vi "relayInternalCommand.vi"(8 "error in (no error)":errorcluster, 11 "DataListenerThisComponent in":refnum<class "DataListenerThisComponent.lvclass">) -> (0 "error out":errorcluster, 3 "DataListenerThisComponent out":refnum<class "DataListenerThisComponent.lvclass">)   [LabVIEW 2015]
uses:
  ComponentTemplateCore/ComponentModel/ComponentModel/DataListener/DataListener.lvclass
  DataListenerThisComponent.lvclass
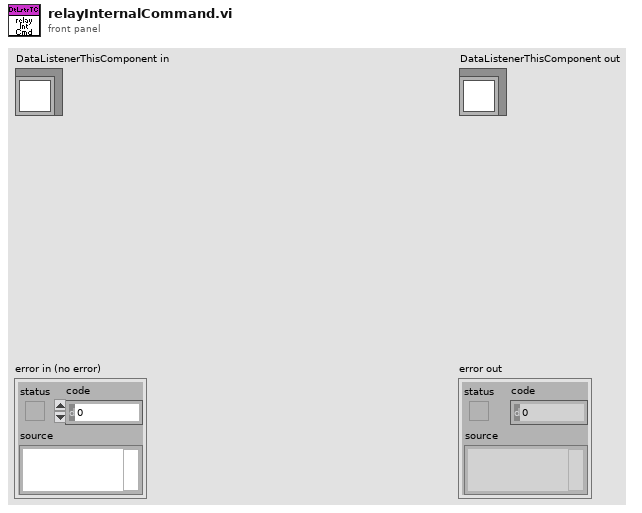
[diagram p1: front panel]
types:
  T1 = typedef "EXATypedefs.lvlib/CommandEvents.ctl" = cluster{"command":refnum<user-event>}
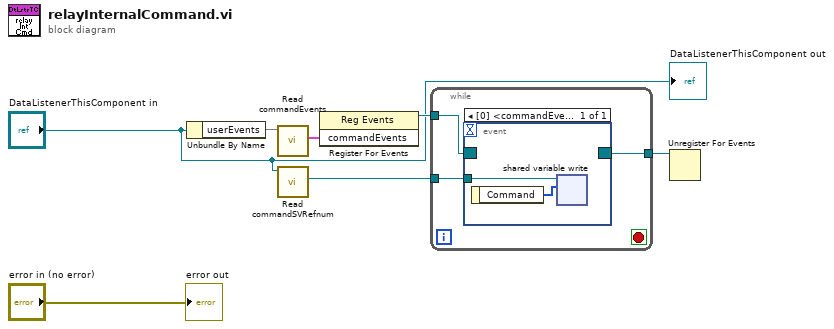
[diagram p0: block diagram]
diagram:
  n1 = Unbundle By Name("DataListenerThisComponent in") -> ("userEvents"=w7)
  n2 = call "Read commandEvents.vi"("UserEventsThisComponent in"=w7) -> ("commandEvents"=w6:T1)  [unwired: 9 in, 1 out]
  n3 = call "Read commandSVRefnum.vi"("DataListener in"="DataListenerThisComponent in") -> ("commandSVRefnum"=w4:refnum<k21>)  [unwired: 9 in, 1 out]
  n4 = register-events(w6) -> (reference out=w5:refnum<event-registration>)  [unwired: 2 in, 1 out]
  n5 = while {
    tunnel: w5 -> [w10]
    tunnel: w4 -> [w9]
    tunnel: [w8] -> w3
    stop <- _ stop-if-true
    n6 = event shown="[0] <commandEvents.command>: User Event" {
      selector: w10 -> [_]
      dyn-events: [_] -> w8
      timeout: _ -> [_]
      tunnel: w9 -> [w11]
      event User Event {
        n7 = event-data() -> ("Command"=w12:u8[])  [unwired: 1 in]
        n8 = shared-variable-write(w11, w12) -> ()  [unwired: 1 in, 2 out]
      }
    }
  }
  n9 = Unregister For Events(event registration refnum=w3) -> ()  [unwired: 1 in, 1 out]
  "error out" <- "error in (no error)"
  "DataListenerThisComponent out" <- "DataListenerThisComponent in"
